vi "Servo Set Pulse Width.vi"   [LabVIEW 2011, in "LVH-LINX.lvlib" / "Servo.lvlib"]
doc: "Set the pulse width of the specified servo channel.\n\nA pulse width of 1500uS is typically the center point of rotation (90 degrees). Most servos can rotate between 1000 and 2000 uS but the actual limits will vary depending on the specific servo.b"
uses:
  Servo.lvlib
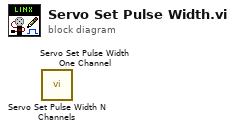
[diagram p0: block diagram]
diagram:
  n1 = call "Servo Set Pulse Width N Channels.vi"() -> ()  [unwired: 10 in, 2 out]
  n2 = call "Servo Set Pulse Width One Channel.vi"() -> ()  [unwired: 10 in, 2 out]
